vi "CheckNumberOfPhases.vi"(8 "error in (no error)":errorcluster, 11 "NHRGridSim in":refnum<class "NHRGridSim.lvclass">) -> (0 "error out":errorcluster, 1 "NumberOfPhases":i32, 2 "Boolean":bool, 3 "NHRGridSim out":refnum<class "NHRGridSim.lvclass">)   [LabVIEW 2018, in "AcPwrPlugins.lvlib" / "NHRGridSim.lvclass"]
uses:
  NHRGridSim.lvclass
  <vilib>/Utility/error.llb/Error Cluster From Error Code.vi
  <vilib>/ErrorRing/Error Ring.xnode
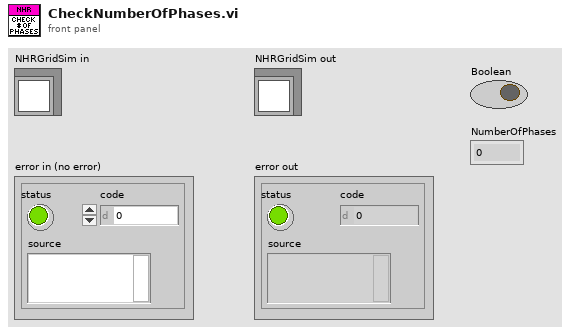
[diagram p1: front panel]
types:
  T1 = cluster{"SlewRates":cluster{"Islew":dbl, "Vslew":dbl, "Pslew":dbl, "FreqSlew":dbl, "AngleABSlew":dbl, "AngleACSlew":dbl}, "Phases":cluster{"Pout (W)":dbl, "Iout (A)":dbl, "PhaseAngle":dbl, "Vout (V)":dbl, "Phase Name":string}[], "Measurement":cluster{"ApertureLength (s)":dbl, "NumberOfSamples":u32}, "Ranges":cluster{"Irange (A)":dbl, "Vrange (V)":dbl}, "Mode":enum8{"One 3-Phase AC", "One AC", "One DC", "Three AC", "Three DC", "One 2-Phase AC and One AC", "One 2-Phase AC and One DC", "Two AC", "One AC and One DC", "Two AC and One DC", "One AC and Two DC", "One DC and One AC", "Two DC"}, "PowerMax":u16, "TransformerRatio":dbl, "Waveshape":dbl[], "Handle":string, "FreqOut (Hz)":dbl, "Connected":bool, "Safety Limits":cluster{"Minimum Voltage (V)":dbl, "Minimum Voltage Time (s)":dbl, "Maximum Voltage (V)":dbl, "Maximum Voltage Time (s)":dbl, "Maximum Source Amps (A)":dbl, "Maximum Source Amps Time (s)":dbl, "Maximum Sink Amps (A)":dbl, "Maximum Sink Amps Time (s)":dbl, "Maximum Source Power (W)":dbl, "Maximum Source Power Time (s)":dbl, "Maximum Sink Power (W)":dbl, "Maximum Sink Power Time (s)":dbl, "Peak Voltage (V)":dbl, "Peak Voltage Enable":bool, "Peak Amps (A)":dbl, "Peak Amps Enable":bool}, "btnIdQuery":bool, "btnReset":bool, "Initialize Timeout (10000 ms)":u32, "Phase (0: All)":i32}[]
  T2 = cluster{"Pout (W)":dbl, "Iout (A)":dbl, "PhaseAngle":dbl, "Vout (V)":dbl, "Phase Name":string}[]
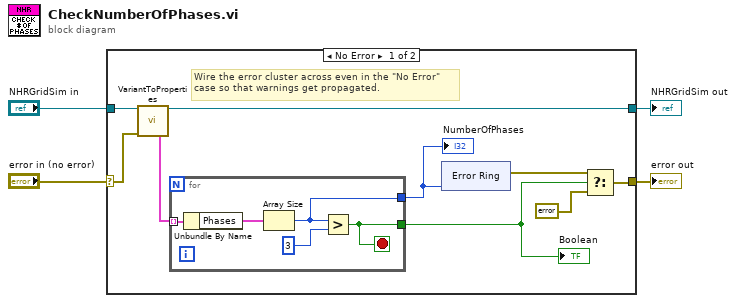
[diagram p0: block diagram]
diagram:
  n1 = case shown="No Error" "error in (no error)" {
    selector: "error in (no error)" -> [w6 w27]
    tunnel: [w9 w27] -> w3
    tunnel: [w7 w26] -> w1
    tunnel: "NHRGridSim in" -> [w8 w26]
    frame No Error {
      # "Wire the error cluster across even in the \"No Error\"\ncase so that warnings get propagated."
      n2 = call "VariantToProperties.vi"("NHRGridSim in"=w8, "error in (no error)"=w6) -> ("NHRGridSim out"=w7:refnum<class "NHRGridSim.lvclass">, "Modules"=w5:T1)  [unwired: 7 in, 5 out]
      n3 = for {
        tunnel: w5 -> [w23] mode=indexing
        tunnel: [w22] -> w10
        tunnel: [w21] -> w13
        stop <- w22 stop-if-true
        n4 = Unbundle By Name(w23) -> ("Phases"=w25:T2)
        n5 = Array Size(array=w25) -> (size(s)=w21:i32)
        n6 = Greater?(x=w21, y=3) -> (0:w22:bool)
      }
      "NumberOfPhases" <- w13
      "Boolean" <- w10
      n7 = xnode "Error Ring"("parameter 0"=w13) -> ("error out"=w12:errorcluster)
      n8 = Select(t=w12, s=w10, f=errorcluster {"status"=FALSE, "code"=0, "source"=""}) -> (s? t:f=w9:errorcluster)
    }
    frame Error {
    }
  }
  "error out" <- w3
  "NHRGridSim out" <- w1
